vi "SetClass - Window Info.vi"(5 "error in (no error)":errorcluster, 7 "Window Info":T1(array[cluster])) -> (19 "error out":errorcluster)   [LabVIEW 2020, in "SPWB.lvclass"]
uses:
  SPWB.lvclass
  API/GSwFormDSP_class/GSwFormDSP.lvclass
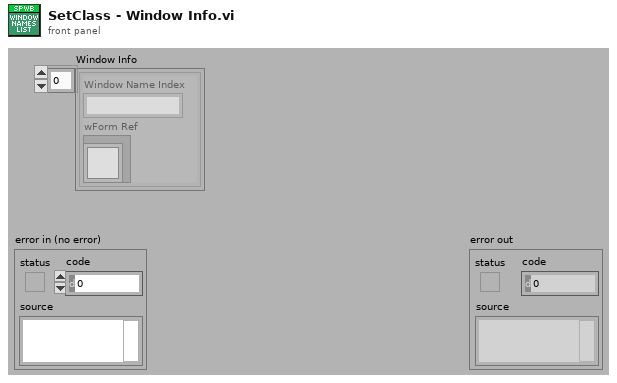
[diagram p1: front panel]
types:
  T1 = cluster{"Window Name Index":string, "wForm Ref":refnum<class "GSwFormDSP.lvclass">}[]
  T2 = typedef "SPWB.lvclass/ClassAttributesRef.ctl" = refnum<data-value>
  T3 = typedef "SPWB.lvclass/ClassAttributes.ctl" = cluster{"Window Info":cluster{"Window Name Index":string, "wForm Ref":refnum<class "GSwFormDSP.lvclass">}[]}
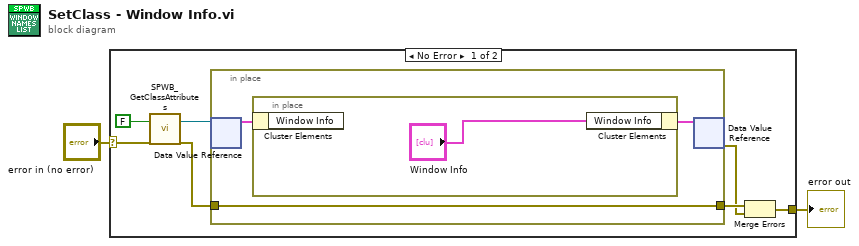
[diagram p0: block diagram]
diagram:
  n1 = case shown="No Error" "error in (no error)" {
    selector: "error in (no error)" -> [w9 w14]
    tunnel: [w6 w14] -> w1
    frame No Error {
      n2 = call "SPWB_GetClassAttributes.vi"("return data? (T)"=FALSE ("return data"), "error in (no error)"=w9) -> ("class attributes ref"=w7:T2, "error out"=w8:errorcluster)  [unwired: 14 in, 2 out]
      n3 = in-place {
        in-place-border: w8 -> [w10]
        in-place-border: [w10] -> w4
        n4 = in-place-dvr #1(w7) -> (w11:T3)  [unwired: 1 out]
        n5 = in-place {
          n6 = in-place-cluster #2(w11) -> ()  [unwired: 1 out]
          n7 = in-place-cluster #2("Window Info"="Window Info") -> (w12:T3)
        }
        n8 = in-place-dvr #1(w12) -> (w3:errorcluster)  [unwired: 1 out]
      }
      n9 = Merge Errors(w4, w3) -> (w6:errorcluster)
    }
    frame Error {
    }
  }
  "error out" <- w1
